vi "QAM Demod.vi"(2 "FFT Downsampled":cdb[](array[numeric]), 3 "QAM Complexity":T1(ring)) -> (0 "QAM Data Symbols":cdb[](array[numeric]), 1 "BitStream Out":i32[](array[numeric]))   [LabVIEW 2018]
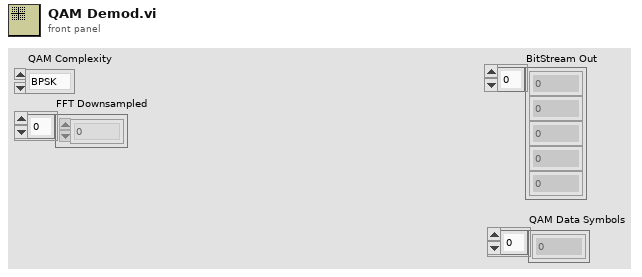
[diagram p1: front panel]
types:
  T1 = enum16{"BPSK", "QPSK", "16-QAM", "64-QAM", "256-QAM"}
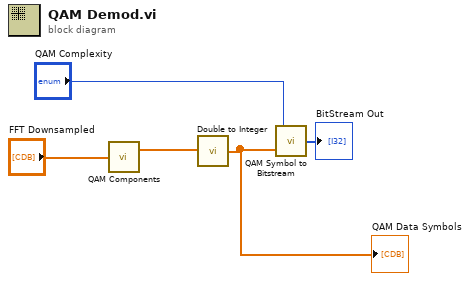
[diagram p0: block diagram]
diagram:
  n1 = call "QAM Components.vi"("FFT Downsampled"="FFT Downsampled") -> ("FFT , Data"=w2:cdb[])  [unwired: 1 out]
  n2 = call "Double to Integer.vi"("DBL Array"=w2) -> ("I32 Array"=w1:cdb[])
  "QAM Data Symbols" <- w1
  n3 = call "QAM Symbol to Bitstream.vi"("Symbol In"=w1, "QAM Complexity"="QAM Complexity") -> ("BitStream Out"=→"BitStream Out":i32[])
